vi "reprTextual.vi"(8 "error in (no error)":errorcluster, 11 "StationKeeping in":refnum<class "StationKeeping.lvclass">) -> (0 "error out":errorcluster, 2 "Description":string, 3 "StationKeeping out":refnum<class "StationKeeping.lvclass">)   [LabVIEW 2011, in "StationKeeping.lvclass"]
uses:
  StationKeeping.lvclass
  StationKeeping.lvclass/StationKeeping.ctl
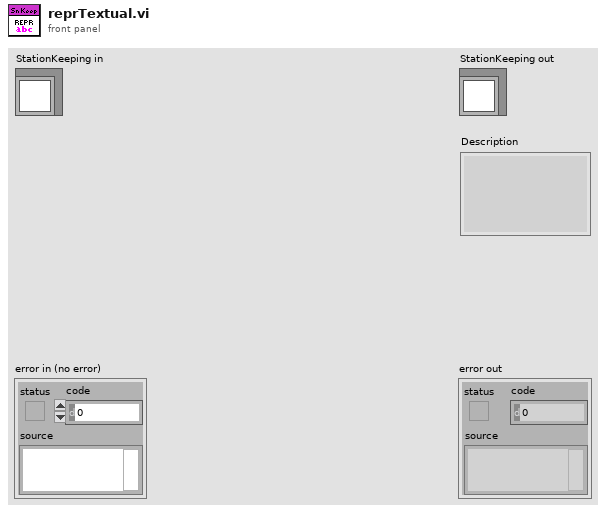
[diagram p1: front panel]
types:
  T1 = typedef "UTM Location.ctl" = cluster{"UTM Zone":dbl, "Hemisphere":enum16{"North", "South"}, "East":dbl, "North":dbl}
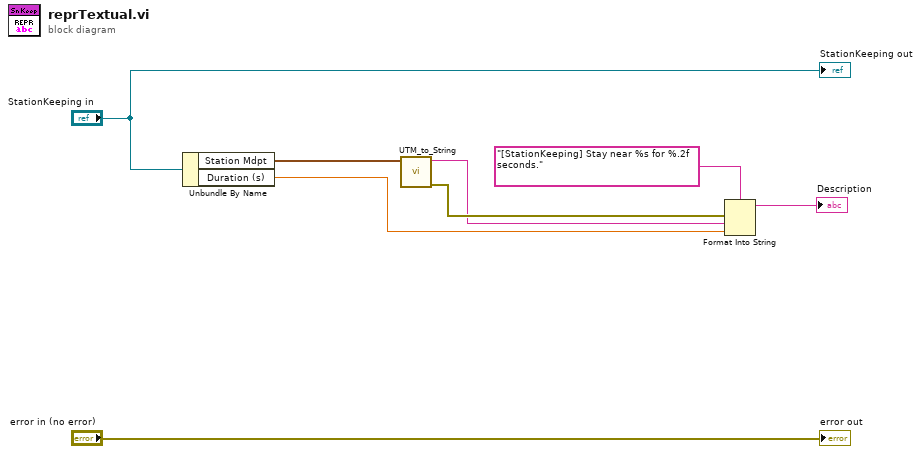
[diagram p0: block diagram]
diagram:
  n1 = Unbundle By Name("StationKeeping in") -> ("Station Mdpt"=w5:T1, "Duration (s)"=w1:dbl)
  n2 = call "UTM_to_String.vi"("UTM Location"=w5) -> ("error out"=w6:errorcluster, "UTM String"=w2:string)  [unwired: 9 in]
  n3 = Format Into String(format string="[StationKeeping] Stay near %s for %.2f seconds.", error in=w6, w2, w1) -> (resulting string=→"Description":string)  [unwired: 1 in, 1 out]
  "error out" <- "error in (no error)"
  "StationKeeping out" <- "StationKeeping in"
